vi "TIFFStream Close.vi"(8 "error in (no error)":errorcluster, 9 "Current and next IFD offset":u32[](array[numeric]), 10 "Image data reference":refnum<data-value>, 11 "File data":T1) -> (0 "error out":errorcluster)   [LabVIEW 2018]
uses:
  kernel32.dll
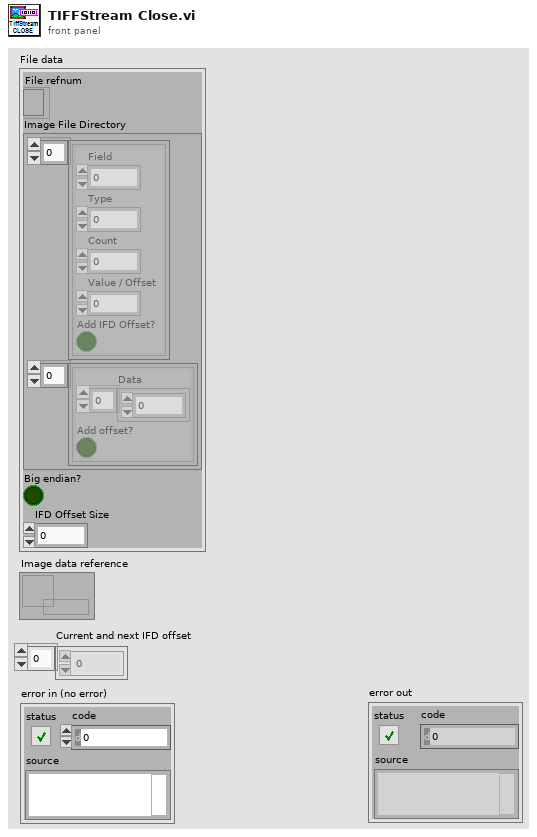
[diagram p1: front panel]
types:
  T1 = cluster{"File refnum":refnum<file>, "Image File Directory":cluster{cluster{"Field":u16, "Type":u16, "Count":u32, "Value / Offset":u32, "Add IFD Offset?":bool}[], cluster{"Data":u32[], "Add offset?":bool}[]}, "Big endian?":bool, "IFD Offset Size":u32}
  T2 = cluster{cluster{"Field":u16, "Type":u16, "Count":u32, "Value / Offset":u32, "Add IFD Offset?":bool}[], cluster{"Data":u32[], "Add offset?":bool}[]}
  T3 = cluster{"Field":u16, "Type":u16, "Count":u32, "Value / Offset":u32, "Add IFD Offset?":bool}[]
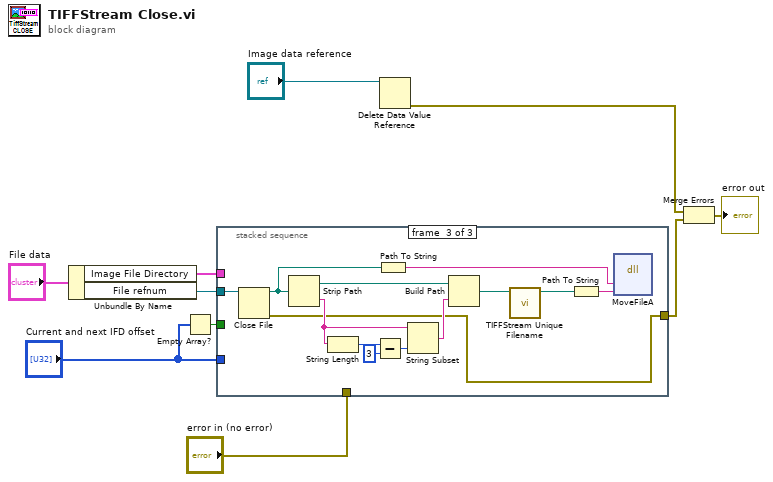
[diagram p0: block diagram]
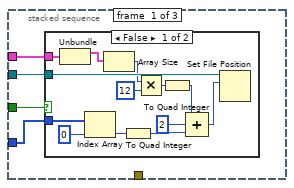
[diagram p2: hidden frame]
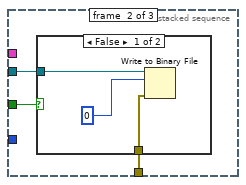
[diagram p4: hidden frame]
diagram:
  n1 = Unbundle By Name("File data") -> ("Image File Directory"=w1:T2, "File refnum"=w8:refnum<file>)
  n2 = Empty Array?(array="Current and next IFD offset") -> (empty?=w2:bool)
  n3 = stacked-sequence {
    tunnel: w8 -> [w14 w30 w46]
    tunnel: [_ _ w36] -> w6
    tunnel: "error in (no error)" -> [_ w29 _]
    tunnel: "Current and next IFD offset" -> [w13 _ _]
    tunnel: w2 -> [w12 w28 _]
    tunnel: w1 -> [w11 _ _]
    frame #0 {
      n4 = case shown="False" w12 {
        tunnel: w14 -> [w27 _]
        tunnel: w13 -> [w23 _]
        tunnel: w11 -> [w21 _]
        frame False {
          n5 = Unbundle(w21) -> (w20:T3)  [unwired: 1 out]
          n6 = Index Array(array=w23, index=0) -> (element=w25:u32)
          n7 = Array Size(array=w20) -> (size(s)=w19:i32)
          n8 = To Quad Integer(1:w25) -> (0:w24:i64)
          n9 = Multiply(x=w19, y=12) -> (x*y=w16:i32)
          n10 = To Quad Integer(1:w16) -> (0:w15:i64)
          n11 = Compound Arithmetic op=ADD(w15, i64 2 ("x"), w24) -> (w22:i64)
          n12 = Set File Position(offset (in bytes) (0)=w22, refnum=w27) -> ()  [unwired: 2 in, 2 out]
        }
        frame True {
        }
      }
    }
    frame #1 {
      n13 = case shown="False" w28 {
        tunnel: w30 -> [w33 _]
        tunnel: w29 -> [w31 _]
        frame False {
          n14 = Write to Binary File(file (use dialog)=w33, data=0, error in=w31) -> ()  [unwired: 3 in, 3 out]
        }
        frame True {
        }
      }
    }
    frame #2 {
      n15 = Close File(refnum=w46) -> (path=w38:path, error out=w36:errorcluster)  [unwired: 1 in]
      n16 = Strip Path(path=w38) -> (stripped path=w41:path, name=w42:string)
      n17 = String Length(string=w42) -> (length=w45:i32)
      n18 = Subtract(x=w45, y=3) -> (x-y=w43:i32)
      n19 = Path To String(path=w38) -> (string=w37:string)
      n20 = String Subset(string=w42, length (rest)=w43) -> (substring=w40:string)  [unwired: 1 in]
      n21 = Build Path(base path=w41, name or relative path=w40) -> (appended path=w35:path)
      n22 = call "TIFFStream Unique Filename.vi"("Path in"=w35) -> ("Unique path out"=w34:path)  [unwired: 10 in]
      n23 = Path To String(path=w34) -> (string=w39:string)
      n24 = dll-call lib="kernel32.dll" fn="MoveFileA"("arg1"=w37, "arg2"=w39) -> ()  [unwired: 6 in, 2 out]
    }
  }
  n25 = Delete Data Value Reference(data value reference="Image data reference") -> (error out=w7:errorcluster)  [unwired: 1 in, 1 out]
  n26 = Merge Errors(w7, w6) -> (→"error out":errorcluster)
